vi "Set Retry Delay.vi"(8 "error in":errorcluster, 10 "Retry Delay":i32=1000 format="%d ms", 11 "Transfer Beginner in":refnum<class "Transfer Beginner.lvclass">) -> (0 "error out":errorcluster, 3 "Transfer Beginner out":refnum<class "Transfer Beginner.lvclass">)   [LabVIEW 2020, in "CANopen.lvlib" / "Transfer Beginner.lvlib" / "Transfer Beginner.lvclass"]
uses:
  Transfer Beginner.lvclass
  Transfer Beginner.lvclass/Transfer Beginner.ctl
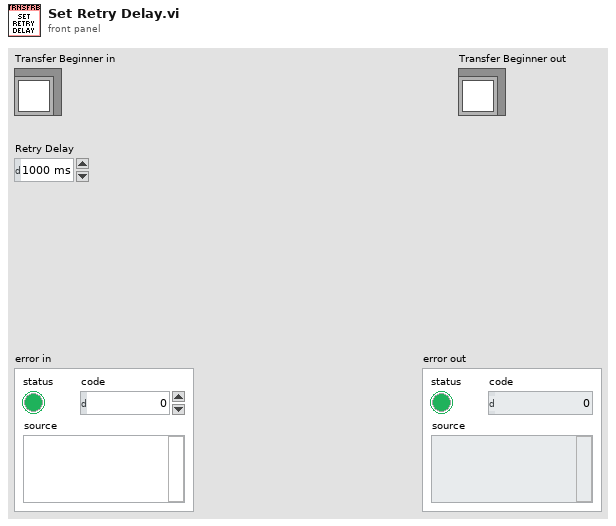
[diagram p1: front panel]
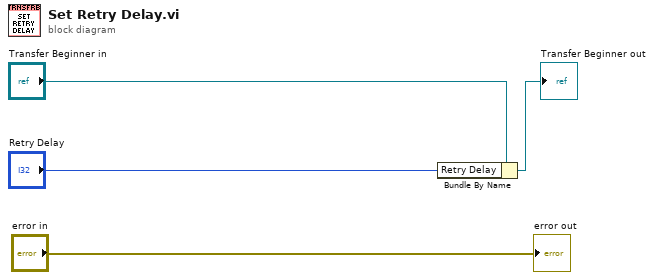
[diagram p0: block diagram]
diagram:
  n1 = Bundle By Name(cluster="Transfer Beginner in", "Retry Delay"="Retry Delay") -> (→"Transfer Beginner out":refnum<class "Transfer Beginner.lvclass">)
  "error out" <- "error in"
